vi "Keithley6487 Open.vi"(3 "VISA resource name":refnum<visa-resource-name>="COM3") -> (0 "Error out":errorcluster, 1 "VISA out":refnum<visa-resource-name>)   [LabVIEW 2018]
uses:
  <vilib>/Instr/_visa.llb/VISA Configure Serial Port (Instr).vi
panel:
  out "Initial Config Read Buffer":string
  in  "Initial Configuration":string="*RST;FORM:ELEM READ;:CURR:RANG:AUTO 0;:CURR:RANG 2E-2;:SOUR:VOLT 0;:SOUR:VOLT:RANG 10;:SOUR:VOLT:ILIM 2.5E-2;:SOUR:VOLT:STAT 1;:SYST:ZCH 0;*IDN?"
  in  "Enable Limits on Auto Range":bool
  in  "Auto Range Limits":string=":RANG:AUTO:ULIM 2.1E-2;LLIM 2.1E-9"
  in  "XON Character":u8=17 format="%.0x"
  in  "XOFF Character":u8=19 format="%.0x"
  in  "Flow Control":u16(ring)=1 items=["None"=0, "XON/XOFF"=1, "RTS/CTS"=2, "DTR/DSR"=4]
  in  "Termination Char\n(0xA = '\\n' = LF)":u8=10 format="%.0x"
  in  "End read on termination character?":bool=TRUE
  in  "Timeout (ms)":u32=1000
  in  "Stop Bits":u16(ring)=10 items=["1.0"=10, "1.5"=15, "2.0"=20]
  in  "Parity":u16(ring) items=["None", "Odd", "Even", "Mark", "Space"]
  in  "Data Bits":u16=8 min=5 max=8 step=1
  in  "Baud Rate":u32=9600
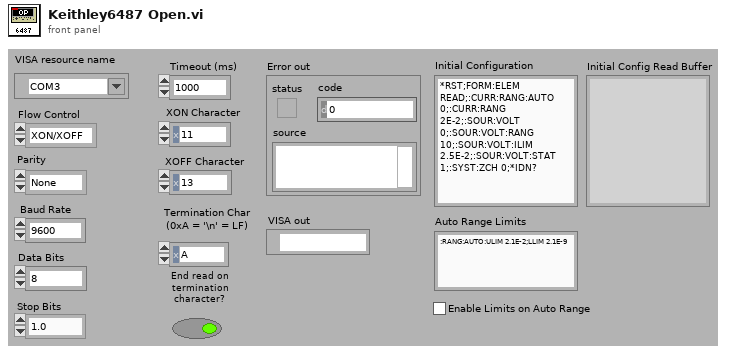
[diagram p1: front panel]
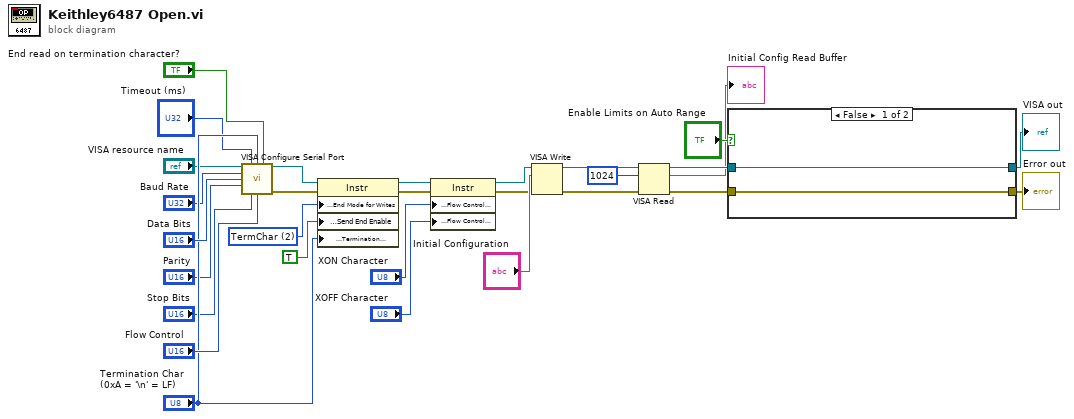
[diagram p0: block diagram]
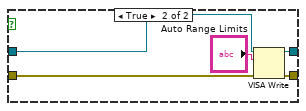
[diagram p2: hidden frame]
diagram:
  w26 = u16 2 items=["None", "LastBit", "TermChar", "Break"] ("Serial Settings:Serial End Mode for Writes")
  n1 = call-poly "VISA Configure Serial Port"("VISA resource name"="VISA resource name", "timeout (10sec)"="Timeout (ms)", "termination char\n(0xA = '\\n' = LF)"="Termination Char\n(0xA = '\\n' = LF)", "Enable Termination\nChar (T)"="End read on termination character?", "baud rate (9600)"="Baud Rate", "data bits (8)"="Data Bits", "parity (0:none)"="Parity", "stop bits (10: 1 bit)"="Stop Bits", "flow control (0:none)"="Flow Control") -> ("VISA resource name out"=w25:refnum<visa-resource-name>, "error out"=w24:errorcluster)  [unwired: 1 in, 4 out]
  n2 = property on="Property Node" class="Instr"(reference=w25, error in=w24, "Serial Settings:End Mode for Writes"=w26, "Message Based Settings:Send End Enable"=TRUE, "Message Based Settings:Termination Character"="Termination Char\n(0xA = '\\n' = LF)") -> (reference out=w28:refnum<visa-resource-name>, error out=w29:errorcluster)
  n3 = property class="Instr"(reference=w28, error in=w29, "Serial Settings:Flow Control XON Character"="XON Character", "Serial Settings:Flow Control XOFF Character"="XOFF Character") -> (reference out=w10:refnum<visa-resource-name>, error out=w9:errorcluster)
  n4 = VISA Write(VISA resource name=w10, write buffer="Initial Configuration", error in (no error)=w9) -> (VISA resource name out=w6:refnum<visa-resource-name>, error out=w4:errorcluster)  [unwired: 1 out]
  n5 = VISA Read(VISA resource name=w6, byte count=u32 1024, error in (no error)=w4) -> (VISA resource name out=w5:refnum<visa-resource-name>, read buffer=→"Initial Config Read Buffer":string, error out=w3:errorcluster)  [unwired: 1 out]
  n6 = case shown="False" "Enable Limits on Auto Range" {
    tunnel: w5 -> [w31 w36]
    tunnel: w3 -> [w30 w35]
    tunnel: [w31 w34] -> w8
    tunnel: [w30 w32] -> w7
    frame False {
    }
    frame True {
      n7 = VISA Write(VISA resource name=w36, write buffer="Auto Range Limits", error in (no error)=w35) -> (VISA resource name out=w34:refnum<visa-resource-name>, error out=w32:errorcluster)  [unwired: 1 out]
    }
  }
  "Error out" <- w7
  "VISA out" <- w8
